vi "Write Priority.vi"(8 "error in":errorcluster, 10 "Priority":i32=1, 11 "synchronous engine configuration in":refnum<class "synchronous engine configuration.lvclass">) -> (0 "error out":errorcluster, 3 "synchronous engine configuration out":refnum<class "synchronous engine configuration.lvclass">)   [LabVIEW 2013, in "synchronous engine configuration.lvclass"]
uses:
  synchronous engine configuration.lvclass
  synchronous engine configuration.lvclass/synchronous engine configuration.ctl
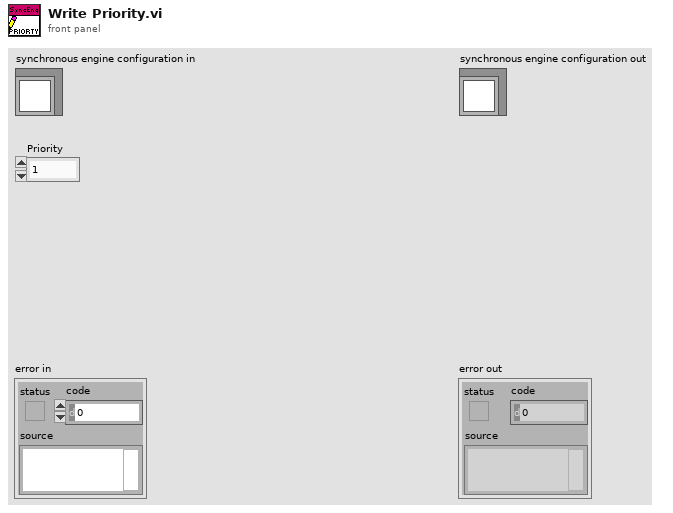
[diagram p1: front panel]
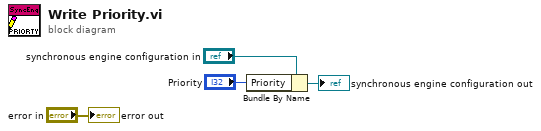
[diagram p0: block diagram]
diagram:
  n1 = Bundle By Name(cluster="synchronous engine configuration in", "Priority"="Priority") -> (→"synchronous engine configuration out":refnum<class "synchronous engine configuration.lvclass">)
  "error out" <- "error in"
